vi "SeriellWriteFPGA.vi"   [LabVIEW 2017]
uses:
  gvboolesch.vi
  <vilib>/rvi/DataTransferAndStorage/Container/XNode/niFpgaContainer.xnode
  <vilib>/eio/EIOMethodNode/EIOMethodNode.xnode
  <vilib>/rvi/eio/common/nirviEmuTemplateMethod_errors.vi
  <vilib>/rvi/interface/RandomDataEmulation/nirviRandomDataFpgaReadWriteTemplate.vi
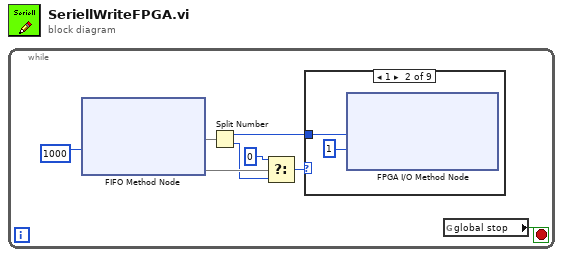
[diagram p0: block diagram]
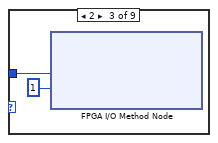
[diagram p3: hidden frame]
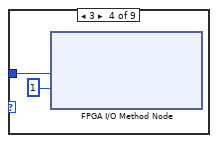
[diagram p4: hidden frame]
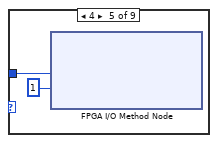
[diagram p5: hidden frame]
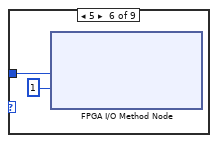
[diagram p6: hidden frame]
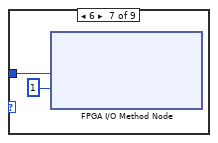
[diagram p7: hidden frame]
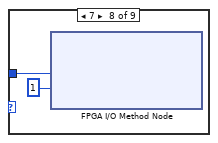
[diagram p8: hidden frame]
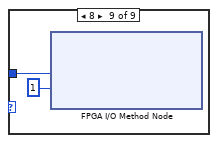
[diagram p9: hidden frame]
diagram:
  n1 = while {
    stop <- w8 stop-if-true
    n2 = xnode ("FIFO Method Node")("Timeout"=1000) -> ("Element"=w3, "Timeout?"=w6)  [unwired: 1 in, 1 out]
    n3 = Split Number(x=w3) -> (hi(x)=w1:u16, lo(x)=w2:u16)
    n4 = Select(t=u8 0, s=w6, f=w2) -> (s? t:f=w5:u8)
    n5 = case shown="1" w5 {
      tunnel: w1 -> [_ w10 w12 w14 w16 w18 w20 w22 w24]
      frame 0, Default {
      }
      frame 1 {
        n6 = xnode "FPGA I/O Method Node"("Data"=w10, "Timeout (ms)"=1) -> ()  [unwired: 1 in, 2 out]
      }
      frame 2 {
        n7 = xnode "FPGA I/O Method Node"("Data"=w12, "Timeout (ms)"=1) -> ()  [unwired: 1 in, 2 out]
      }
      frame 3 {
        n8 = xnode "FPGA I/O Method Node"("Data"=w14, "Timeout (ms)"=1) -> ()  [unwired: 1 in, 2 out]
      }
      frame 4 {
        n9 = xnode "FPGA I/O Method Node"("Data"=w16, "Timeout (ms)"=1) -> ()  [unwired: 1 in, 2 out]
      }
      frame 5 {
        n10 = xnode "FPGA I/O Method Node"("Data"=w18, "Timeout (ms)"=1) -> ()  [unwired: 1 in, 2 out]
      }
      frame 6 {
        n11 = xnode "FPGA I/O Method Node"("Data"=w20, "Timeout (ms)"=1) -> ()  [unwired: 1 in, 2 out]
      }
      frame 7 {
        n12 = xnode "FPGA I/O Method Node"("Data"=w22, "Timeout (ms)"=1) -> ()  [unwired: 1 in, 2 out]
      }
      frame 8 {
        n13 = xnode "FPGA I/O Method Node"("Data"=w24, "Timeout (ms)"=1) -> ()  [unwired: 1 in, 2 out]
      }
    }
    n14 = global read "gvboolesch.vi" "global stop"() -> (w8:bool)
  }
